vi "iterate_image.vi"(8 "error in (no error)":errorcluster, 11 "DL090215DataCollection in":refnum<class "DataCollectionDL090215.lvclass">) -> (0 "error out":errorcluster, 3 "DL090215DataCollection out":refnum<class "DataCollectionDL090215.lvclass">)   [LabVIEW 2010, in "DataCollectionDL090215.lvclass"]
uses:
  DataCollectionDL090215.lvclass
  DataCollectionDL090215.lvclass/DataCollectionDL090215.ctl
  common/classes/ErrorController/ErrorController/class_data.vi
  common/classes/ErrorController/ErrorController/ErrorController.lvclass
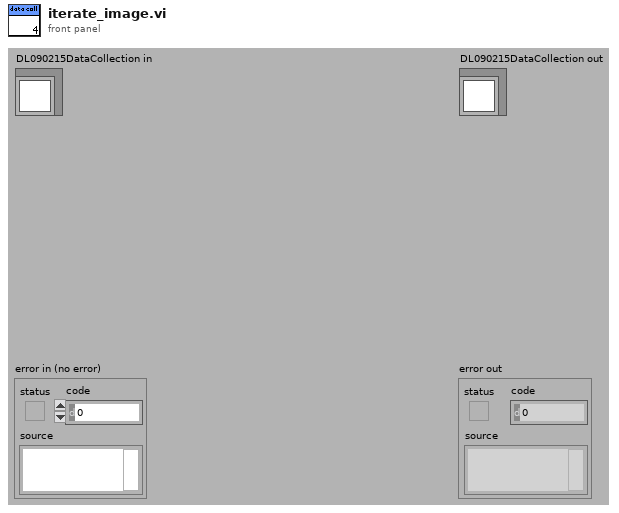
[diagram p1: front panel]
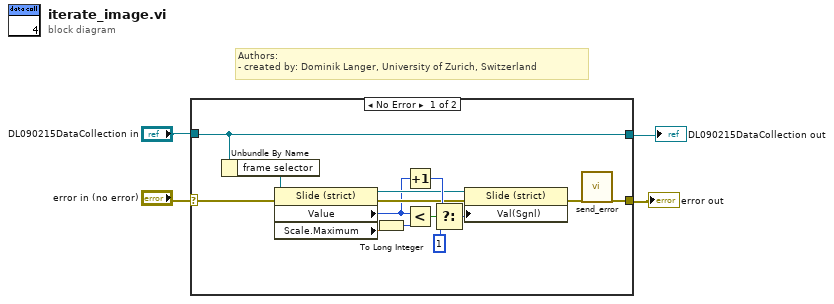
[diagram p0: block diagram]
diagram:
  # "Authors: \n- created by: Dominik Langer, University of Zurich, Switzerland"
  n1 = case shown="No Error" "error in (no error)" {
    selector: "error in (no error)" -> [w18 w20]
    tunnel: [w6 w20] -> w3
    tunnel: [w8 w19] -> w1
    tunnel: "DL090215DataCollection in" -> [w8 w19]
    frame No Error {
      n2 = Unbundle By Name(w8) -> ("frame selector"=w5:refnum<vi>)
      n3 = property class="Slide (strict)"(reference=w5, error in=w18) -> (reference out=w12:refnum<vi>, error out=w13:errorcluster, "Value"=w11:i32, "Scale.Maximum"=w10:dbl)
      n4 = To Long Integer(number=w10) -> (32bit integer=w9:i32)
      n5 = Increment(x=w11) -> (x+1=w15:i32)
      n6 = Less?(x=w11, y=w9) -> (x < y?=w14:bool)
      n7 = Select(t=w15, s=w14, f=1) -> (s? t:f=w17:i32)
      n8 = property class="Slide (strict)"(reference=w12, error in=w13, "Val(Sgnl)"=w17) -> (error out=w7:errorcluster)  [unwired: 1 out]
      n9 = call "send_error.vi"("error in (no error)"=w7) -> ("error out"=w6:errorcluster)  [unwired: 10 in]
    }
    frame Error {
    }
  }
  "error out" <- w3
  "DL090215DataCollection out" <- w1
